vi "run_simulation.vi"(8 "inputSpecs":string, 9 "Run":refnum<vi>) -> (0 "OK":bool, 1 "TMP Filepath":path, 2 "standard error":string, 3 "standard output":string)   [LabVIEW 2019]
uses:
  <vilib>/Utility/sysdir.llb/System Directory Type.ctl
  lib/libBioGasLabViewWrapper.so
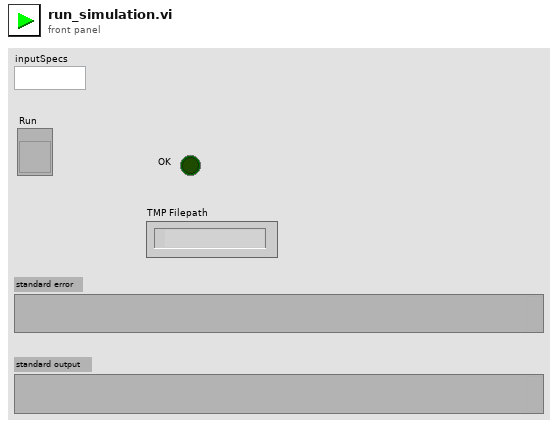
[diagram p1: front panel]
types:
  T1 = enum8{"Enabled", "Disabled", "Disabled and Grayed Out"}
  T2 = typedef "System Directory Type.ctl" = i32
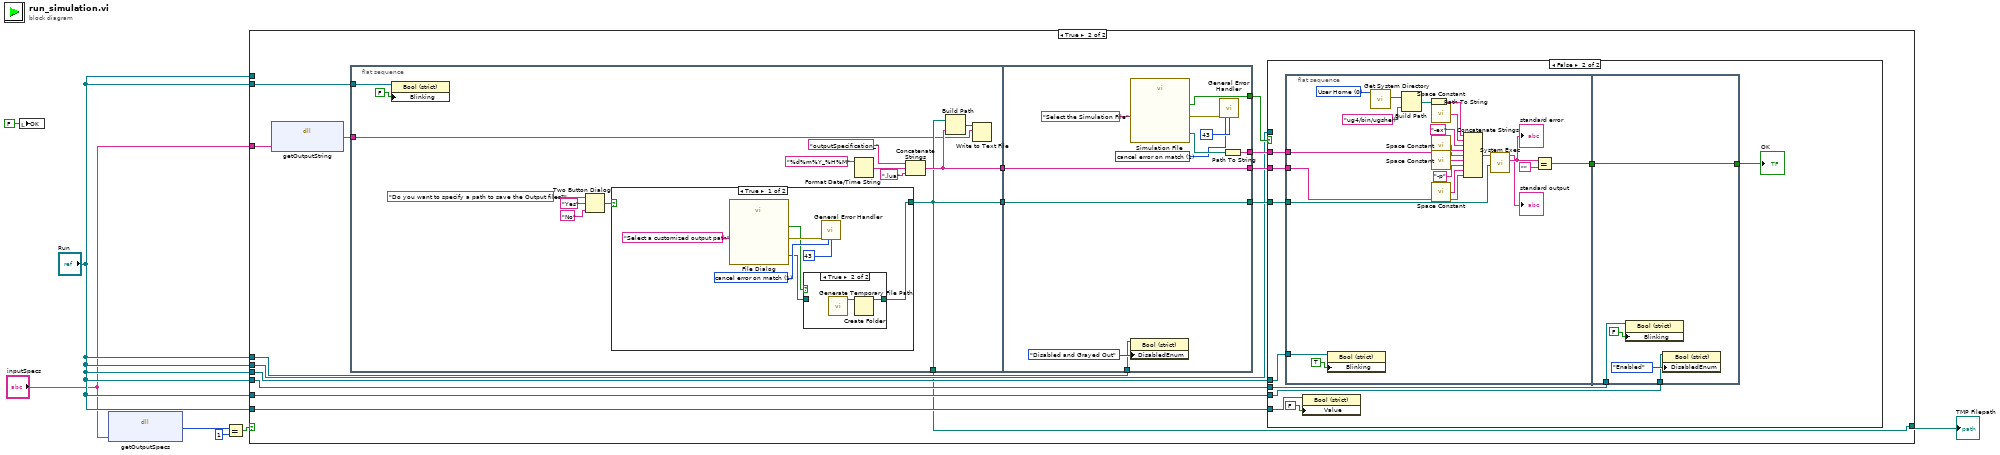
[diagram p0: block diagram]
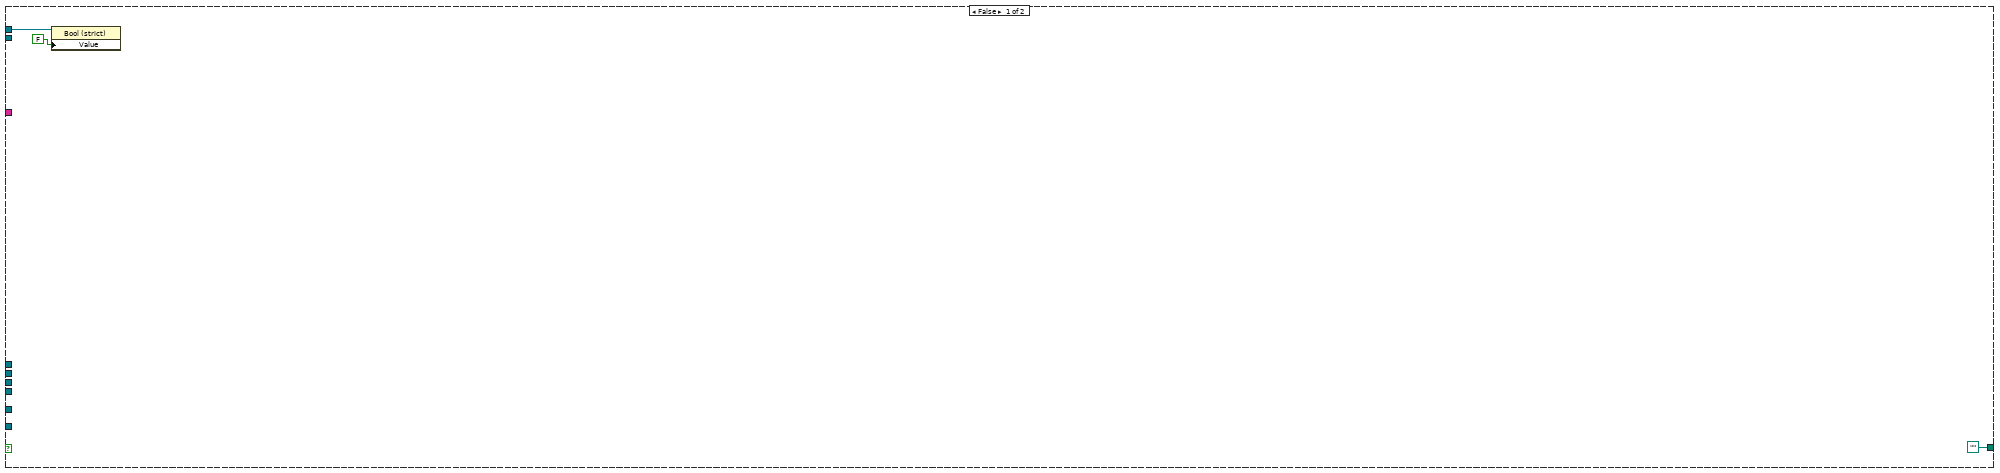
[diagram p2: hidden frame]
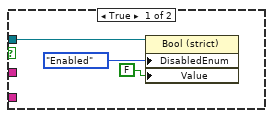
[diagram p3: hidden frame]
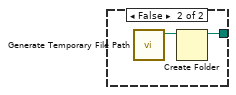
[diagram p5: hidden frame]
diagram:
  n1 = local write "OK"(FALSE ("OK")) -> ()
  n2 = dll-call lib="home/paul/Schreibtisch/Biogas_LabView_Wrapper/lib/libBioGasLabViewWrapper.so" fn="getOutputSpecs"("inputSpecs"="inputSpecs") -> ("isValid"=w1:i32)  [unwired: 4 in, 2 out]
  n3 = Equal?(x=w1, y=1) -> (x = y?=w2:bool)
  n4 = case shown="True" w2 {
    tunnel: "inputSpecs" -> [_ w26]
    tunnel: "Run" -> [w9 _]
    tunnel: "Run" -> [_ w20]
    tunnel: "Run" -> [_ w19]
    tunnel: "Run" -> [_ w18]
    tunnel: "Run" -> [_ w17]
    tunnel: "Run" -> [_ w16]
    tunnel: "Run" -> [_ w15]
    tunnel: "Run" -> [_ w14]
    tunnel: [path "" w13] -> w6
    frame False {
      n5 = property on="Property Node" class="Bool (strict)"(reference=w9, "Value"=FALSE ("Run")) -> ()  [unwired: 1 in, 2 out]
    }
    frame True {
      n6 = dll-call lib="home/paul/Schreibtisch/Biogas_LabView_Wrapper/lib/libBioGasLabViewWrapper.so" fn="getOutputString"("inputSpecs"=w26) -> ("outputString"=w25:string)  [unwired: 4 in, 2 out]
      n7 = flat-sequence {
        tunnel: w25 -> [w66]
        tunnel: [w67] -> w12
        tunnel: [w69] -> w11
        tunnel: w20 -> [w78]
        tunnel: [w67] -> w13
        tunnel: w12 -> [w95]
        tunnel: w11 -> [w96]
        tunnel: [w97] -> w24
        tunnel: [w96] -> w23
        tunnel: [w95] -> w22
        tunnel: [w94] -> w21
        tunnel: w19 -> [w92]
        frame #0 {
          n8 = property on="Property Node" class="Bool (strict)"(reference=w78, "Blinking"=FALSE) -> ()  [unwired: 1 in, 2 out]
          n9 = Two Button Dialog(message="Do you want to specify a path to save the Output files?", 1:"No" ("F button name (\"Cancel\")"), 2:"Yes" ("T button name (\"OK\")")) -> (T button?=w74:bool)
          n10 = case shown="True" w74 {
            tunnel: [w82 w90] -> w67
            frame True {
              w84 = 1 items=["no exception", "cancel error on match", "set error on match"] ("[exception action] (none:0)")
              n11 = call "File Dialog"("prompt"="Select a customized output path") -> ("selected path"=w83:path, "cancelled"=w81:bool, "error out"=w86:errorcluster)  [unwired: 11 in, 1 out]
              n12 = case shown="True" w81 {
                tunnel: w83 -> [w87 _]
                tunnel: [w87 w88] -> w82
                frame False {
                }
                frame True {
                  n13 = call <vilib>:"Generate Temporary File Path.vi"() -> ("Unique Temporary File Path"=w89:path)  [unwired: 10 in, 1 out]
                  n14 = Create Folder(path (use dialog)=w89) -> (created path=w88:path)  [unwired: 2 in, 2 out]
                }
              }
              n15 = call <vilib>:"General Error Handler.vi"("error in (no error)"=w86, "[exception action] (none:0)"=w84, "[exception code]"=43) -> ()  [unwired: 8 in, 5 out]
            }
            frame False {
              n16 = call <vilib>:"Generate Temporary File Path.vi"() -> ("Unique Temporary File Path"=w91:path)  [unwired: 10 in, 1 out]
              n17 = Create Folder(path (use dialog)=w91) -> (created path=w90:path)  [unwired: 2 in, 2 out]
            }
          }
          n18 = Format Date/Time String(time format string (%c)="%d%m%Y_%H%M") -> (date/time string=w71:string)  [unwired: 2 in]
          n19 = Concatenate Strings("outputSpecification_" ("string"), w71, ".lua" ("string")) -> (w69:string)
          n20 = Build Path(base path=w67, name or relative path=w69) -> (appended path=w68:path)
          n21 = Write to Text File(file (use dialog)=w68, text=w66) -> ()  [unwired: 2 in, 3 out]
        }
        frame #1 {
          w99 = 1 items=["no exception", "cancel error on match", "set error on match"] ("[exception action] (none:0)")
          n22 = call "Simulation File"("prompt"="Select the Simulation File") -> ("selected path"=w101:path, "cancelled"=w97:bool, "error out"=w98:errorcluster)  [unwired: 11 in, 1 out]
          n23 = property on="Property Node" class="Bool (strict)"(reference=w92, "DisabledEnum"=T1."Disabled and Grayed Out" ("Disabled")) -> ()  [unwired: 1 in, 2 out]
          n24 = call <vilib>:"General Error Handler.vi"("error in (no error)"=w98, "[exception action] (none:0)"=w99, "[exception code]"=43) -> ()  [unwired: 8 in, 5 out]
          n25 = Path To String(path=w101) -> (string=w94:string)
        }
      }
      n26 = case shown="False" w24 {
        tunnel: w23 -> [_ w37]
        tunnel: w22 -> [_ w38]
        tunnel: w21 -> [_ w36]
        tunnel: w18 -> [w28 _]
        tunnel: w17 -> [_ w34]
        tunnel: w16 -> [_ w33]
        tunnel: w15 -> [_ w32]
        tunnel: w14 -> [_ w31]
        frame True {
          n27 = property on="Property Node" class="Bool (strict)"(reference=w28, "DisabledEnum"=T1."Enabled" ("Disabled"), "Value"=FALSE) -> ()  [unwired: 1 in, 2 out]
        }
        frame False {
          n28 = flat-sequence {
            tunnel: w38 -> [w47]
            tunnel: w37 -> [w46]
            tunnel: w36 -> [w45]
            tunnel: [w42] -> w35
            tunnel: w33 -> [w41]
            tunnel: [w65] -> w30
            tunnel: w35 -> [w65]
            tunnel: w32 -> [w62]
            tunnel: w31 -> [w61]
            frame #0 {
              w51 = T2 0 items=["User Home"=0, "User Desktop"=1, "User Documents"=2, "User Application Data"=3, "User Preferences"=4, "User Temporary"=5, "Public Documents"=6, "Public Application Data"=7, "Public Preferences"=8, "Public Cache"=13, "System Core Libraries"=9, "System Installed Libraries"=10, "Application Files"=11, "Boot Volume Root"=12] ("system directory type")
              n29 = property on="Property Node" class="Bool (strict)"(reference=w41, "Blinking"=TRUE) -> ()  [unwired: 1 in, 2 out]
              n30 = call <vilib>:"Get System Directory.vi"("system directory type"=w51) -> ("system directory"=w59:path)  [unwired: 10 in]
              n31 = Build Path(base path=w59, name or relative path="ug4/bin/ugshell") -> (appended path=w57:path)
              n32 = Path To String(path=w57) -> (string=w53:string)
              n33 = call <vilib>:"Space Constant.vi"() -> ("String"=w54:string)
              n34 = call <vilib>:"Space Constant.vi"() -> ("String"=w55:string)
              n35 = call <vilib>:"Space Constant.vi"() -> ("String"=w56:string)
              n36 = call <vilib>:"Space Constant.vi"() -> ("String"=w60:string)
              n37 = Concatenate Strings(w53, w54, "-ex" ("command line"), w55, w45, w56, "-p" ("command line"), w60, w46) -> (w58:string)
              n38 = call <vilib>:"System Exec.vi"("working directory"=w47, "command line"=w58) -> ("standard error"=w43:string, "standard output"=→"standard output":string)  [unwired: 6 in, 2 out]
              "standard error" <- w43
              n39 = Equal?(x=w43, y="") -> (x = y?=w42:bool)
            }
            frame #1 {
              n40 = property on="Property Node" class="Bool (strict)"(reference=w61, "Blinking"=FALSE) -> ()  [unwired: 1 in, 2 out]
              n41 = property on="Property Node" class="Bool (strict)"(reference=w62, "DisabledEnum"=T1."Enabled" ("Disabled")) -> ()  [unwired: 1 in, 2 out]
            }
          }
          n42 = property class="Bool (strict)"(reference=w34, "Value"=FALSE ("Run")) -> ()  [unwired: 1 in, 2 out]
          "OK" <- w30
        }
      }
    }
  }
  "TMP Filepath" <- w6
